vi "Index_Problem_Crossconnection_Solving-1.vi"(0 "[IN] Used Index":i32, 1 "[IN] Defined Index":i32, 2 "[IN] 1st Index for Deletion":i32, 3 "[IN] 2nd Index for Deletion":i32, 4 "[IN] Is it first step?":bool) -> (5 "[OUT] Index of Track wi\nth Point For Deletion":i32)   [LabVIEW 2013]
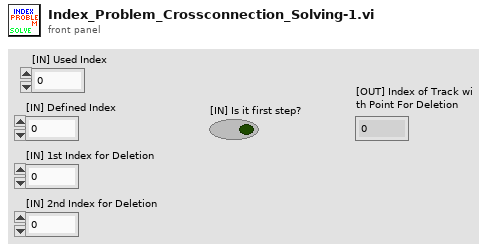
[diagram p1: front panel]
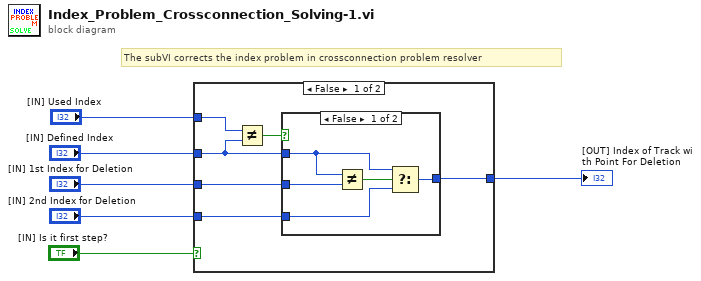
[diagram p0: block diagram]
diagram:
  # "The subVI corrects the index problem in crossconnection problem resolver"
  n1 = case shown="False" "[IN] Is it first step?" {
    tunnel: "[IN] Defined Index" -> [w10 w19]
    tunnel: "[IN] Used Index" -> [w12 _]
    tunnel: "[IN] 1st Index for Deletion" -> [w9 _]
    tunnel: "[IN] 2nd Index for Deletion" -> [w8 _]
    tunnel: [w7 w19] -> w1
    frame False {
      n2 = Not Equal?(x=w12, y=w10) -> (x != y?=w11:bool)
      n3 = case shown="False" w11 {
        tunnel: w10 -> [w15 w18]
        tunnel: w9 -> [w17 _]
        tunnel: w8 -> [w14 _]
        tunnel: [w13 w18] -> w7
        frame False {
          n4 = Not Equal?(x=w15, y=w17) -> (x != y?=w16:bool)
          n5 = Select(t=w15, s=w16, f=w14) -> (s? t:f=w13:i32)
        }
        frame True {
        }
      }
    }
    frame True {
    }
  }
  "[OUT] Index of Track wi\nth Point For Deletion" <- w1
